vi "playback shoulder.vi"(4 "Home":bool, 5 "Rewind":bool, 7 "Playback":bool, 8 "Taper Limit":dbl=1.0, 9 "Playback allow":bool=TRUE, 10 "Encoder Recording Data":cluster{dbl, u32}[](array[cluster])=[{0.0, 20}, {0.0, 41}, {0.0, 60}, {0.0, 80}, {0.0, 100}, {0.0, 120}, {0.0, 141}, {0.0, 160}, {0.0, 180}, {0.0, 200}, {0.0, 220}, {0.0, 244}, {0.0, 263}, {0.0, 283}, {0.0, 303}, {0.0, 322}, {0.0, 343}, {0.0, 364}, {0.0, 385}, {0.0, 406}, {0.0, 421}, {0.0, 442}, {0.0, 465}, {0.0, 486}, {0.0, 510}, {0.0, 527}, {0.0, 547}, {0.0, 567}, {0.0, 586}, {0.0, 606}, {0.0, 626}, {0.0, 649}, {0.0, 669}, {0.0, 689}, {0.0, 709}, {0.0, 730}, {0.0, 750}, {0.0, 769}, {0.0, 789}, {0.0, 809}, {0.0, 830}, {0.0, 849}, {0.0, 870}, {0.0, 891}, {0.0, 911}, {0.0, 931}, {0.0, 953}, {0.0, 974}, {0.0, 993}, {0.0, 1013}, {0.0, 1032}, {0.0, 1052}, {0.0, 1073}, {0.0, 1093}, {0.0, 1114}, {0.0, 1134}, {0.0, 1155}, {0.0, 1174}, {0.0, 1194}, {0.0, 1214}, {0.0, 1235}, {0.0, 1255}, {0.0, 1275}, {0.0, 1297}, {0.0, 1317}, {0.0, 1337}, {0.0, 1357}, {0.0, 1379}, {0.0, 1399}, {0.0, 1417}, {0.0, 1438}, {0.0, 1458}, {0.0, 1479}, {0.0, 1499}, {0.0, 1519}, {0.0, 1540}, {0.0, 1560}, {0.0, 1579}, {0.0, 1600}, {0.0, 1619}, {0.0, 1639}, {0.0, 1660}, {0.0, 1679}, {0.0, 1699}, {0.0, 1720}, {0.0, 1741}, {0.0, 1760}, {0.0, 1787}, {0.0, 1801}, {0.0, 1823}, {0.0, 1841}, {0.0, 1864}, {0.0, 1884}, {0.0, 1904}, {0.0, 1925}, {0.0, 1945}, {0.0, 1966}, {0.0, 1986}, {0.0, 2006}, {0.0, 2028}, {0.0, 2047}, {0.0, 2068}, {0.0, 2087}, {0.0, 2107}, {0.0, 2128}, {0.0, 2147}, {0.0, 2167}, {0.0, 2189}, {0.0, 2208}, {0.0, 2227}, {0.0, 2248}, {0.0, 2268}, {0.0, 2288}, {0.0, 2308}, {0.0, 2329}, {0.0, 2348}, {0.0, 2369}, {0.0, 2389}, {0.0, 2408}, {0.0, 2429}, {0.0, 2448}, {-0.25, 2469}, {-1.0, 2488}, {-2.0, 2508}, {-2.75, 2529}, {-4.0, 2550}, {-4.5, 2570}, {-4.75, 2590}, {-5.0, 2610}, {-5.0, 2630}, {-5.25, 2651}, {-6.0, 2674}, {-7.0, 2693}, {-7.0, 2712}, {-7.25, 2734}, {-7.25, 2755}, {-7.25, 2775}, {-7.25, 2795}, {-7.5, 2815}, {-7.5, 2836}, {-8.0, 2855}, {-8.25, 2875}, {-8.75, 2896}, {-9.5, 2917}, {-9.75, 2937}, {-10.25, 2957}, {-10.75, 2977}, {-11.0, 2997}, {-11.5, 3016}, {-12.25, 3037}, {-13.25, 3058}, {-14.0, 3077}, {-15.0, 3097}, {-16.25, 3117}, {-17.5, 3137}, {-18.75, 3157}, {-20.0, 3178}, {-21.5, 3198}, {-23.0, 3218}, {-24.5, 3238}, {-26.0, 3258}, {-27.5, 3278}, {-28.75, 3298}, {-30.25, 3318}, {-31.25, 3339}, {-32.0, 3359}, {-32.25, 3380}, {-32.75, 3400}, {-33.25, 3419}, {-34.5, 3444}, {-35.0, 3461}, {-35.5, 3481}, {-36.0, 3501}, {-36.25, 3521}, {-36.75, 3541}, {-37.25, 3560}, {-38.0, 3581}, {-39.0, 3600}, {-40.25, 3620}, {-41.75, 3641}, {-43.25, 3661}, {-45.25, 3680}, {-48.0, 3704}, {-49.75, 3720}, {-52.0, 3741}, {-54.75, 3762}, {-57.5, 3782}, {-61.0, 3806}, {-63.5, 3822}, {-67.0, 3844}, {-70.25, 3865}, {-73.0, 3886}, {-75.75, 3904}, {-78.5, 3926}, {-81.0, 3945}, {-83.5, 3965}, {-86.25, 3986}, {-89.0, 4006}, {-91.75, 4026}, {-94.75, 4046}, {-97.75, 4066}, {-101.25, 4087}, {-105.5, 4108}, {-109.5, 4128}, {-113.75, 4149}, {-118.5, 4169}, {-123.5, 4190}, {-127.75, 4209}, {-132.75, 4229}, {-137.75, 4249}, {-142.5, 4269}, {-147.25, 4289}, {-151.75, 4309}, {-156.25, 4329}, {-160.75, 4349}, {-165.25, 4369}, {-169.5, 4389}, {-173.75, 4409}, {-178.0, 4429}, {-182.25, 4449}, {-186.5, 4469}, {-191.25, 4490}, {-195.75, 4510}, {-200.25, 4529}, {-205.0, 4549}, {-210.25, 4570}, {-215.25, 4590}, {-220.25, 4609}, {-225.75, 4629}, {-230.75, 4650}, {-235.75, 4669}, {-241.25, 4690}, {-246.5, 4710}, {-251.75, 4731}, {-257.0, 4751}, {-261.75, 4770}, {-266.75, 4791}, {-271.75, 4811}, {-276.5, 4830}, {-282.0, 4854}, {-286.5, 4873}, {-292.0, 4894}, {-296.25, 4910}, {-301.25, 4931}, {-306.25, 4950}, {-311.25, 4970}, {-317.0, 4993}, {-322.25, 5013}, {-327.25, 5033}, {-332.25, 5053}, {-337.25, 5073}, {-342.25, 5093}, {-346.5, 5112}, {-351.5, 5133}, {-356.0, 5153}, {-360.5, 5173}, {-365.0, 5193}, {-369.5, 5213}, {-373.75, 5233}, {-378.75, 5256}, {-383.25, 5277}, {-387.5, 5295}, {-391.5, 5314}, {-396.0, 5334}, {-400.5, 5354}, {-405.25, 5376}, {-410.0, 5396}, {-414.25, 5415}, {-419.0, 5435}, {-423.5, 5454}, {-428.0, 5474}, {-432.5, 5495}, {-437.0, 5516}, {-441.25, 5534}, {-445.75, 5555}, {-450.25, 5576}, {-454.5, 5594}, {-458.5, 5615}, {-462.5, 5634}, {-466.5, 5654}, {-471.25, 5677}, {-475.75, 5698}, {-479.5, 5717}, {-484.0, 5738}, {-488.25, 5758}, {-492.25, 5779}, {-496.75, 5799}, {-500.75, 5820}, {-504.75, 5839}, {-509.0, 5859}, {-513.0, 5878}, {-517.25, 5899}, {-521.25, 5918}, {-525.5, 5938}, {-529.5, 5958}, {-533.75, 5979}, {-537.75, 5999}, {-541.5, 6019}, {-545.5, 6039}, {-549.25, 6059}, {-553.25, 6079}, {-556.75, 6098}, {-560.75, 6120}, {-564.25, 6138}, {-568.0, 6159}, {-571.75, 6179}, {-575.5, 6200}, {-579.0, 6219}, {-582.75, 6240}, {-586.5, 6261}, {-590.0, 6280}, {-593.75, 6300}, {-597.5, 6321}, {-600.75, 6339}, {-604.5, 6360}, {-608.25, 6381}, {-611.75, 6399}, {-615.25, 6419}, {-619.0, 6439}, {-623.25, 6462}, {-626.75, 6480}, {-630.5, 6500}, {-634.25, 6519}, {-638.25, 6540}, {-642.0, 6559}, {-646.5, 6581}, {-650.5, 6600}, {-654.75, 6620}, {-658.75, 6639}, {-663.0, 6660}, {-667.25, 6679}, {-671.75, 6699}, {-676.25, 6720}, {-680.75, 6740}, {-685.25, 6761}, {-690.0, 6782}, {-694.25, 6802}, {-699.0, 6822}, {-704.25, 6847}, {-709.0, 6867}, {-713.25, 6887}, {-717.75, 6907}, {-722.25, 6927}, {-727.0, 6949}, {-731.75, 6970}, {-736.5, 6991}, {-741.0, 7011}, {-745.75, 7031}, {-750.75, 7051}, {-756.25, 7074}, {-760.5, 7092}, {-765.0, 7111}, {-770.75, 7133}, {-774.75, 7150}, {-780.25, 7173}, {-785.25, 7194}, {-790.25, 7214}, {-795.0, 7235}, {-799.75, 7255}, {-804.75, 7276}, {-809.0, 7295}, {-814.0, 7316}, {-819.0, 7338}, {-823.5, 7357}, {-828.0, 7377}, {-832.5, 7398}, {-837.0, 7419}, {-841.25, 7438}, {-845.75, 7459}, {-850.25, 7480}, {-854.5, 7500}, {-858.75, 7521}, {-863.0, 7541}, {-867.5, 7563}, {-871.5, 7582}, {-875.75, 7603}, {-880.0, 7624}, {-884.0, 7644}, {-888.25, 7666}, {-892.5, 7687}, {-896.0, 7704}, {-900.0, 7725}, {-903.5, 7744}, {-907.75, 7765}, {-911.5, 7786}, {-915.5, 7806}, {-918.75, 7825}, {-923.0, 7845}, {-926.75, 7865}, {-930.25, 7886}, {-933.75, 7907}, {-937.5, 7928}, {-940.75, 7947}, {-944.0, 7968}, {-947.25, 7990}, {-949.75, 8006}, {-953.0, 8027}, {-956.0, 8048}, {-958.75, 8068}, {-961.25, 8087}, {-964.0, 8108}, {-966.5, 8128}, {-969.0, 8148}, {-971.0, 8167}, {-973.75, 8190}, {-975.75, 8208}, {-978.0, 8230}, {-980.0, 8250}, {-981.75, 8269}, {-984.0, 8291}, {-986.0, 8312}, {-988.0, 8332}, {-989.5, 8349}, {-991.5, 8373}, {-992.75, 8391}, {-994.0, 8410}, {-995.5, 8431}, {-996.75, 8451}, {-998.0, 8474}, {-999.25, 8494}, {-1000.25, 8514}, {-1001.5, 8535}, {-1002.5, 8557}, {-1003.5, 8577}, {-1004.75, 8595}, {-1006.0, 8615}, {-1007.25, 8634}, {-1008.75, 8657}, {-1010.0, 8676}, {-1011.5, 8697}, {-1013.0, 8717}, {-1014.25, 8736}, {-1015.5, 8756}, {-1016.75, 8777}, {-1017.25, 8798}, {-1017.25, 8817}, {-1017.5, 8837}, {-1017.5, 8857}, {-1017.75, 8880}, {-1018.0, 8895}, {-1018.5, 8918}, {-1019.25, 8937}, {-1020.25, 8957}, {-1021.25, 8979}, {-1021.5, 9006}, {-1021.5, 9018}, {-1021.75, 9042}, {-1022.0, 9057}, {-1022.5, 9078}, {-1023.75, 9106}, {-1024.5, 9120}, {-1026.0, 9139}, {-1027.75, 9159}, {-1029.75, 9179}, {-1031.75, 9199}, {-1034.5, 9220}, {-1036.75, 9239}, {-1039.75, 9259}, {-1042.75, 9278}, {-1045.75, 9299}, {-1049.5, 9319}, {-1052.75, 9338}, {-1055.75, 9358}, {-1058.5, 9378}, {-1061.25, 9399}, {-1063.5, 9418}, {-1066.25, 9438}, {-1068.75, 9458}, {-1071.0, 9479}, {-1073.25, 9498}, {-1075.5, 9519}, {-1077.5, 9538}, {-1079.75, 9559}, {-1082.25, 9582}, {-1084.75, 9603}, {-1087.25, 9621}, {-1090.25, 9644}, {-1093.0, 9662}, {-1096.5, 9685}, {-1099.5, 9705}, {-1102.25, 9723}, {-1105.5, 9745}, {-1108.5, 9764}, {-1112.75, 9790}, {-1115.75, 9809}, {-1118.75, 9830}, {-1121.75, 9851}, {-1124.5, 9870}, {-1127.25, 9890}, {-1130.0, 9909}, {-1132.75, 9931}, {-1135.25, 9949}, {-1138.0, 9970}, {-1140.75, 9991}, {-1143.0, 10009}, {-1145.5, 10029}, {-1148.25, 10050}, {-1151.5, 10073}, {-1154.0, 10090}, {-1157.0, 10110}, {-1159.75, 10130}, {-1163.0, 10150}, {-1166.25, 10172}, {-1170.0, 10194}, {-1173.25, 10215}, {-1176.25, 10235}, {-1179.25, 10254}, {-1182.25, 10275}, {-1185.5, 10297}, {-1188.0, 10315}, {-1190.75, 10336}, {-1193.5, 10356}, {-1196.0, 10376}, {-1198.25, 10395}, {-1200.75, 10416}, {-1202.75, 10437}, {-1205.0, 10456}, {-1207.0, 10476}, {-1209.0, 10497}, {-1211.0, 10517}, {-1213.0, 10536}, {-1215.0, 10556}, {-1216.75, 10577}, {-1218.75, 10597}, {-1220.5, 10617}, {-1222.5, 10638}, {-1224.0, 10658}, {-1225.75, 10678}, {-1227.25, 10699}, {-1229.0, 10720}, {-1230.25, 10738}, {-1232.0, 10759}, {-1233.5, 10780}, {-1235.0, 10799}, {-1236.5, 10819}, {-1238.0, 10839}, {-1239.25, 10858}, {-1240.75, 10879}, {-1242.5, 10901}, {-1243.75, 10919}, {-1245.5, 10940}, {-1247.0, 10960}, {-1248.5, 10979}, {-1250.25, 11000}, {-1251.75, 11020}, {-1253.25, 11041}, {-1254.75, 11060}, {-1256.5, 11081}, {-1257.75, 11099}, {-1259.75, 11123}, {-1261.0, 11140}, {-1262.25, 11159}, {-1263.75, 11180}, {-1265.0, 11200}, {-1266.75, 11220}, {-1268.0, 11239}, {-1269.75, 11259}, {-1271.25, 11280}, {-1272.75, 11299}, {-1274.5, 11320}, {-1276.25, 11340}, {-1278.0, 11364}, {-1279.5, 11381}, {-1281.25, 11401}, {-1283.25, 11424}, {-1284.5, 11441}, {-1286.0, 11462}, {-1287.5, 11485}, {-1288.25, 11500}, {-1289.75, 11521}, {-1290.75, 11540}, {-1291.75, 11563}, {-1292.75, 11581}, {-1293.75, 11601}, {-1294.5, 11621}, {-1295.5, 11643}, {-1296.25, 11661}, {-1297.25, 11682}, {-1298.25, 11704}, {-1299.0, 11724}, {-1300.25, 11744}, {-1301.25, 11764}, {-1302.75, 11783}, {-1304.0, 11802}], 11 "Hardware In":T5={"Motor Selection"="Shoulder", "EncoderDevRef"={"DevStatus"={"status"=FALSE, "code"=0, "source"=""}, "EncoderIndex"=enum."Enc 1", "CounterIndex"=enum."Invalid", "DistancePerCount"=1.0, "Decoding Type"=enum."4x"}}) -> (0 "Encoder Distance PB":dbl)   [LabVIEW 2017]
uses:
  <vilib>/Rock Robotics/WPI/Encoder/WPI_EncoderDevRef.ctl
  <vilib>/Rock Robotics/SystemInterfaces/Encoder/FPGA_EncoderIdx.ctl
  <vilib>/Rock Robotics/SystemInterfaces/Counter/FPGA_CounterCtrSystemIndex.ctl
  <vilib>/Rock Robotics/WPI/Encoder/WPI_EncoderType.ctl
  <vilib>/Rock Robotics/WPI/Utilities/WPI_GetSetVariantRefNum.vi
  <vilib>/addons/control/pid/pid.llb/PID (DBL).vi
  <vilib>/Rock Robotics/WPI/RobotDrive/WPI_RobotDriveArcadeDrive_Standard(NoSaturation).vi
  <vilib>/addons/control/pid/NI_PID_pid.lvlib
panel:
  out "Initial Encoder Position":dbl=-58.0
  out "Waveform Chart":cluster{dbl, dbl}(graph)={0.0, -2.0}
  in  "Playback PID gains":T6={"proportional gain (Kc)"=-0.015, "integral time (Ti, min)"=0.014, "derivative time (Td, min)"=0.0} {"derivative time (Td, min)" format="%.8f"; "integral time (Ti, min)" format="%.8f"; "proportional gain (Kc)" format="%.8f"}
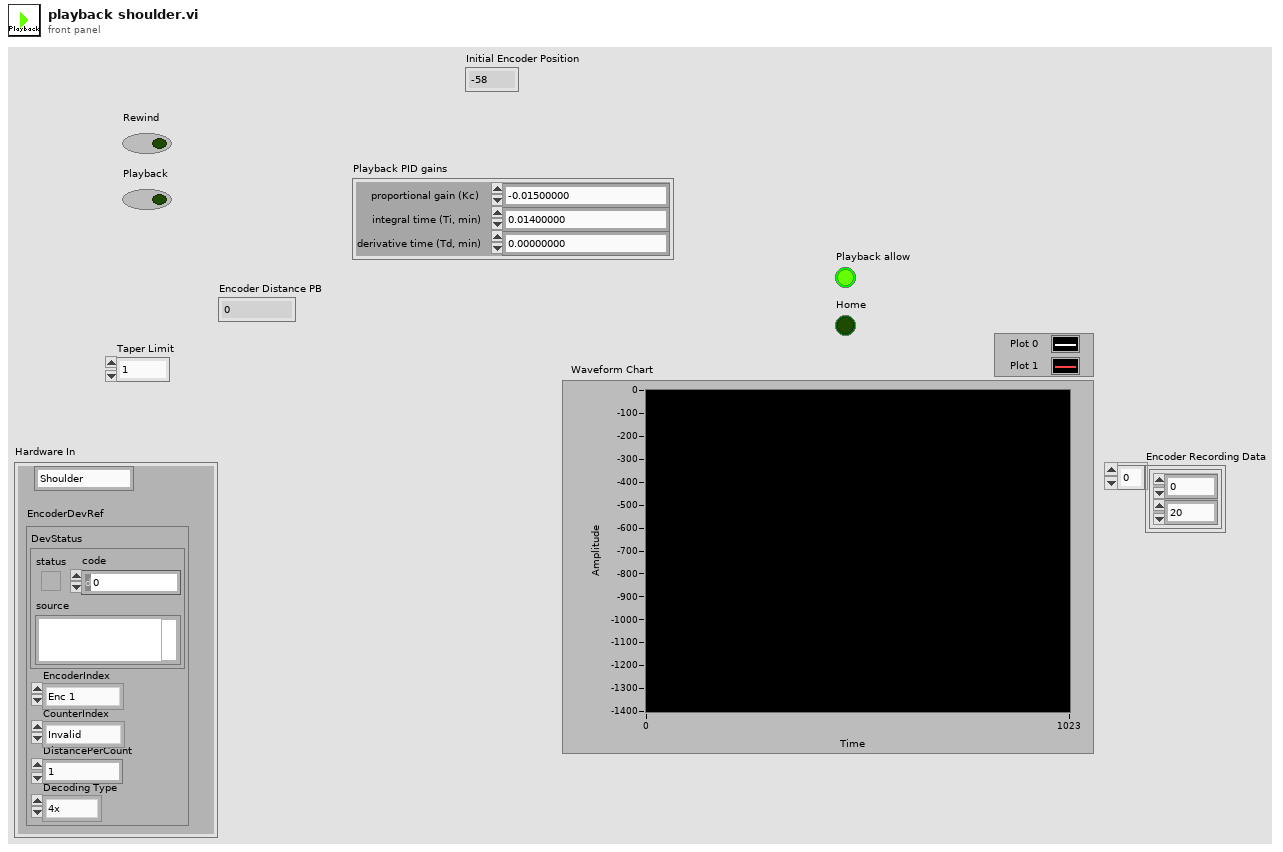
[diagram p1: front panel]
types:
  T1 = typedef "WPI_EncoderDevRef.ctl" = cluster{"DevStatus":errorcluster, "EncoderIndex":T2, "CounterIndex":T3, "DistancePerCount":dbl, "Decoding Type":T4}
  T2 = typedef "FPGA_EncoderIdx.ctl" = enum8{"Enc 0", "Enc 1", "Enc 2", "Enc 3", "Enc 4", "Enc 5", "Enc 6", "Enc 7", "Invalid"}
  T3 = typedef "FPGA_CounterCtrSystemIndex.ctl" = enum8{"Ctr 0", "Ctr 1", "Ctr 2", "Ctr 3", "Ctr 4", "Ctr 5", "Ctr 6", "Ctr 7", "Invalid"}
  T4 = typedef "WPI_EncoderType.ctl" = enum16{"1x", "2x", "4x"}
  T5 = cluster{"Motor Selection":string, "EncoderDevRef":T1}
  T6 = cluster{"proportional gain (Kc)":dbl, "integral time (Ti, min)":dbl, "derivative time (Td, min)":dbl}
  T7 = typedef "WPI_RobotDriveDevRef.ctl" = cluster{"DevStatus":errorcluster, "Motors[]":T8[], "Square Inputs":bool, "Max Output":dbl}
  T8 = typedef "WPI_MotorControlDeviceRef.ctl" = cluster{"DeviceStatus":errorcluster, "Type":T9, "PWM":cluster{"PWM Channel":T10, "DeadBand":T11}, "CAN":cluster{"Device Number":u8, "SetOutput VI Ref":variant, "GetOutput VI Ref":variant, "Enable VI Ref":variant, "Disable VI Ref":variant, "Data":variant}, "Invert":bool, "DIO PWM":cluster{"PWM \"Enable\" Channel":T10, "DIOChannel":T12, "PWM Rate":dbl}}
  T9 = typedef "WPI_MotorControlType.ctl" = enum16{"PWM", "CAN", "DIO PWM"}
  T10 = typedef "FPGA_DIOPWMChannel.ctl" = enum8{"PWM 0", "PWM 1", "PWM 2", "PWM 3", "PWM 4", "PWM 5", "PWM 6", "PWM 7", "PWM 8", "PWM 9", "PWM MXP 0", "PWM MXP 1", "PWM MXP 2", "PWM MXP 3", "PWM MXP 4", "PWM MXP 5", "PWM MXP 6", "PWM MXP 7", "PWM MXP 8", "PWM MXP 9", "Invalid"}
  T11 = typedef "WPI_PWMDeadband.ctl" = cluster{"Name":string, "maxPositivePwm":i32, "minPositivePwm":i32, "centerPwm":i32, "maxNegativePwm":i32, "minNegativePwm":i32, "angularRange":u16}
  T12 = typedef "FPGA_DIOChannel.ctl" = enum8{"DIO 0", "DIO 1", "DIO 2", "DIO 3", "DIO 4", "DIO 5", "DIO 6", "DIO 7", "DIO 8", "DIO 9", "DIO MXP 0", "DIO MXP 1", "DIO MXP 2", "DIO MXP 3", "DIO MXP 4", "DIO MXP 5", "DIO MXP 6", "DIO MXP 7", "DIO MXP 8", "DIO MXP 9", "DIO MXP 10", "DIO MXP 11", "DIO MXP 12", "DIO MXP 13", "DIO MXP 14", "DIO MXP 15", "SPI Port CS1", "SPI Port CS2", "SPI Port CS3", "SPI Port MISO", "SPI Port MOSI", "Invalid"}
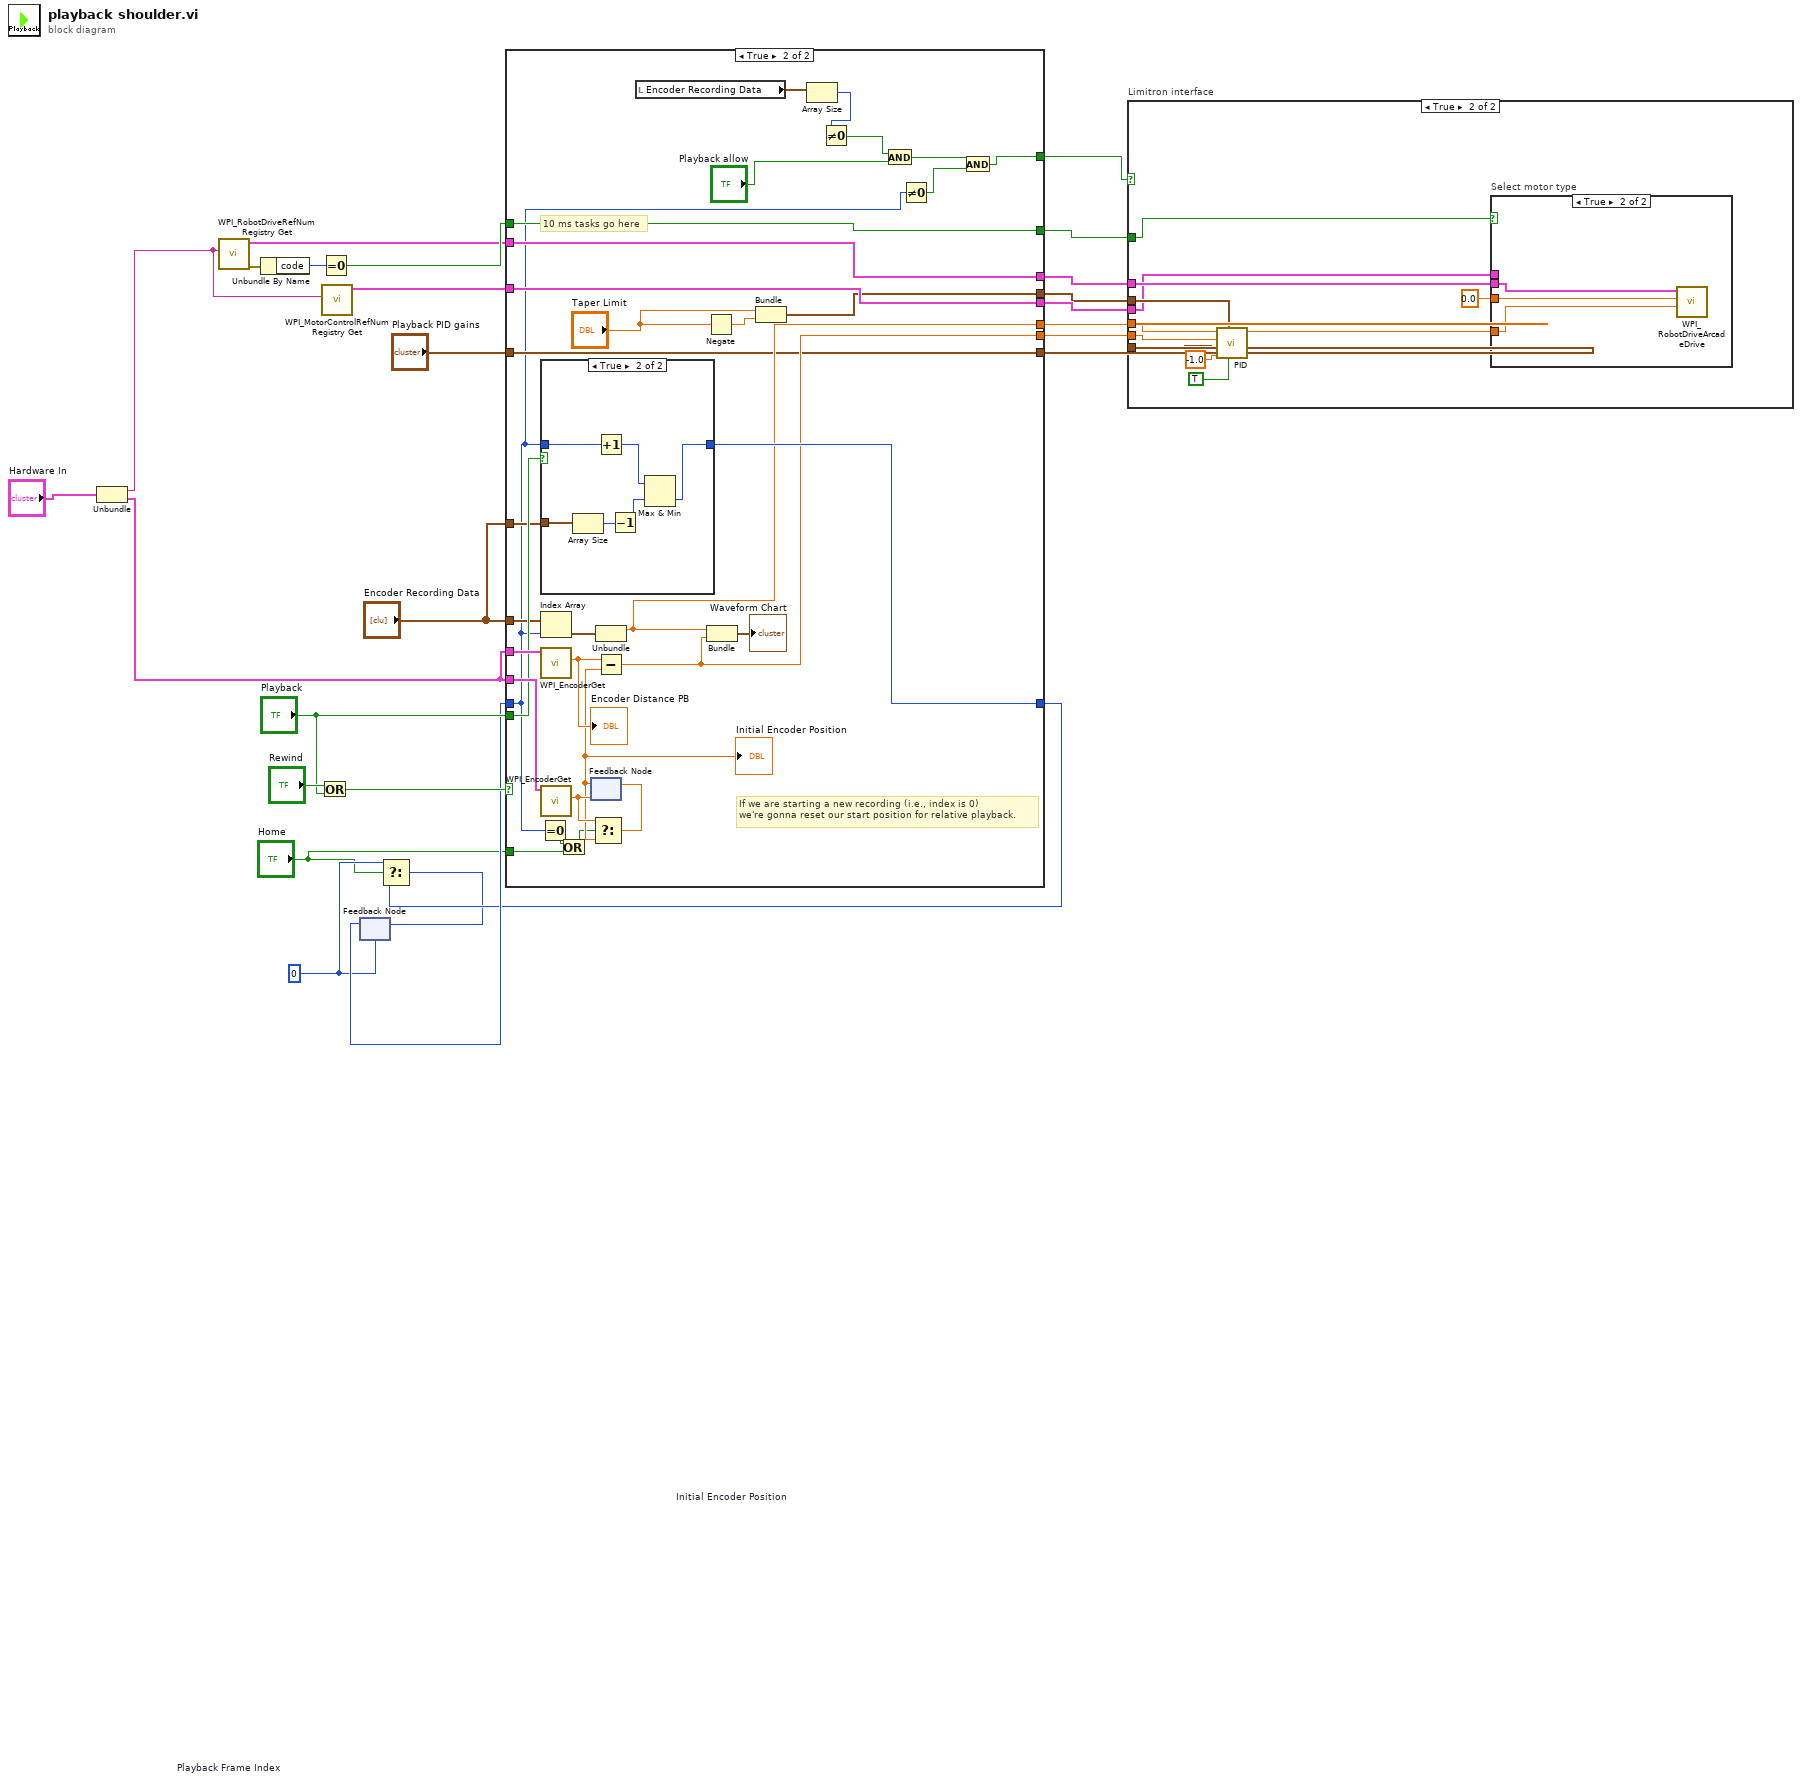
[diagram p0: block diagram]
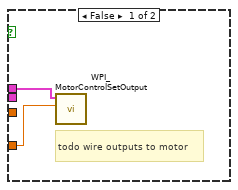
[diagram p3: hidden frame]
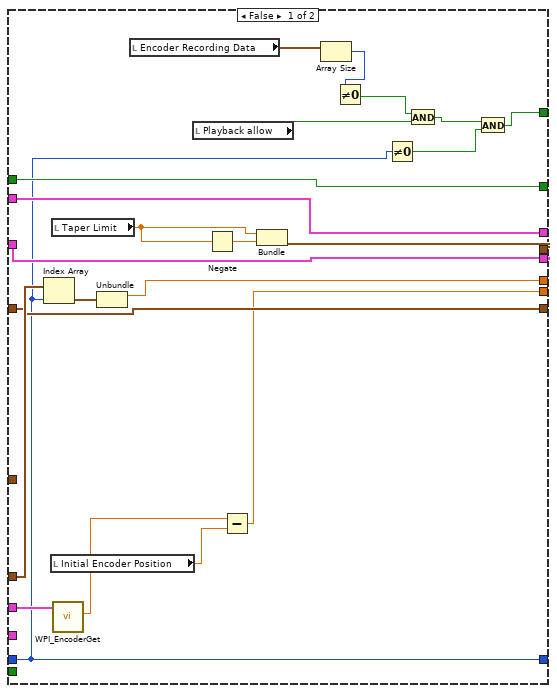
[diagram p4: hidden frame]
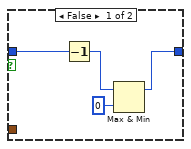
[diagram p5: hidden frame]
diagram:
  w15 = 0 ("index")
  n1 = Unbundle("Hardware In") -> ("Motor Selection"=w11:string, "EncoderDevRef"=w10:T1)
  n2 = call <vilib>:"WPI_RobotDriveRefNum Registry Get.vi"("refnum name"=w11) -> ("error out"=w25:errorcluster, "RobotDriveDevRef"=w23:T7)  [unwired: 1 in, 8 out]
  n3 = Unbundle By Name(w25) -> ("code"=w26:i32)
  n4 = Or(x="Rewind", y="Playback") -> (x .or. y?=w21:bool)
  n5 = Equal To 0?(x=w26) -> (x = 0?=w24:bool)
  n6 = call <vilib>:"WPI_MotorControlRefNum Registry Get.vi"("refnum name"=w11) -> ("MotorControlDevRef"=w19:T8)  [unwired: 9 in, 1 out]
  n7 = feedback #1 "Playback Frame Index"(w15) -> (w18:i32)
  n8 = case shown="True" w21 {
    tunnel: w10 -> [_ w80]
    tunnel: w10 -> [w34 w79]
    tunnel: w24 -> [w44 w67]
    tunnel: w23 -> [w43 w66]
    tunnel: "Playback" -> [_ w78]
    tunnel: w19 -> [w42 w65]
    tunnel: "Encoder Recording Data" -> [w48 w72]
    tunnel: w18 -> [w27 w52]
    tunnel: [w27 w71] -> w16
    tunnel: "Playback PID gains" -> [w40 w61]
    tunnel: "Encoder Recording Data" -> [_ w68]
    tunnel: [w44 w67] -> w9
    tunnel: [w43 w66] -> w8
    tunnel: [w42 w65] -> w7
    tunnel: [w41 w64] -> w6
    tunnel: [w31 w63] -> w5
    tunnel: [w39 w62] -> w4
    tunnel: [w40 w61] -> w3
    tunnel: [w28 w54] -> w2
    tunnel: "Home" -> [_ w49]
    frame False {
      n9 = Index Array(array=w48, index=w27) -> (element=w47:cluster{dbl, u32})
      n10 = local read "Initial Encoder Position"() -> (w32:dbl)
      n11 = local read "Taper Limit"() -> (w45:dbl)
      n12 = call <vilib>:"WPI_EncoderGet.vi"("EncoderDevRef"=w34) -> ("Distance"=w33:dbl)  [unwired: 5 in, 5 out]
      n13 = Unbundle(w47) -> (w41:dbl)  [unwired: 1 out]
      n14 = local read "Encoder Recording Data"() -> (w35:cluster{dbl, u32}[])
      n15 = local read "Playback allow"() -> (w36:bool)
      n16 = Negate(x=w45) -> (-x=w46:dbl)
      n17 = Subtract(x=w33, y=w32) -> (x-y=w31:dbl)
      n18 = Bundle("Taper Limit"=w45, w46) -> (w39:cluster{"Taper Limit":dbl, dbl})  [unwired: 1 in]
      n19 = Array Size(array=w35) -> (size(s)=w38:i32)
      n20 = Not Equal To 0?(x=w38) -> (x != 0?=w37:bool)
      n21 = Not Equal To 0?(x=w27) -> (x != 0?=w29:bool)
      n22 = And(x=w37, y=w36) -> (x .and. y?=w30:bool)
      n23 = And(x=w30, y=w29) -> (x .and. y?=w28:bool)
    }
    frame True {
      # "If we are starting a new recording (i.e., index is 0)\nwe're gonna reset our start position for relative playback."
      # "10 ms tasks go here"
      n24 = Equal To 0?(x=w52) -> (x = 0?=w50:bool)
      n25 = case shown="True" w78 {
        tunnel: [w81 w88] -> w71
        tunnel: w52 -> [w84 w90]
        tunnel: w68 -> [_ w87]
        frame False {
          n26 = Decrement(x=w84) -> (x-1=w82:i32)
          n27 = Max & Min(x=w82, y=0) -> (max(x,y)=w81:i32)  [unwired: 1 out]
        }
        frame True {
          n28 = Array Size(array=w87) -> (size(s)=w86:i32)
          n29 = Increment(x=w90) -> (x+1=w89:i32)
          n30 = Decrement(x=w86) -> (x-1=w85:i32)
          n31 = Max & Min(x=w89, y=w85) -> (min(x,y)=w88:i32)  [unwired: 1 out]
        }
      }
      n32 = Index Array(array=w72, index=w52) -> (element=w73:cluster{dbl, u32})
      n33 = call <vilib>:"WPI_EncoderGet.vi"("EncoderDevRef"=w79) -> ("Distance"=w77:dbl)  [unwired: 5 in, 5 out]
      "Encoder Distance PB" <- w77
      n34 = call <vilib>:"WPI_EncoderGet.vi"("EncoderDevRef"=w80) -> ("Distance"=w70:dbl)  [unwired: 5 in, 5 out]
      n35 = Or(x=w50, y=w49) -> (x .or. y?=w51:bool)
      n36 = feedback #2 "Initial Encoder Position"(w70) -> (w69:dbl)
      "Initial Encoder Position" <- w69
      n37 = Select(t=w70, s=w51, f=w69) -> (s? t:f=w56:dbl)
      n38 = feedback-in #2(w56) -> ()
      n39 = Unbundle(w73) -> (w64:dbl)  [unwired: 1 out]
      n40 = Subtract(x=w77, y=w69) -> (x-y=w63:dbl)
      n41 = local read "Encoder Recording Data"() -> (w59:cluster{dbl, u32}[])
      n42 = Negate(x="Taper Limit") -> (-x=w75:dbl)
      n43 = Bundle(w64, w63) -> (→"Waveform Chart":cluster{dbl, dbl})  [unwired: 1 in]
      n44 = Bundle("Taper Limit"="Taper Limit", w75) -> (w62:cluster{"Taper Limit":dbl, dbl})  [unwired: 1 in]
      n45 = Array Size(array=w59) -> (size(s)=w60:i32)
      n46 = Not Equal To 0?(x=w60) -> (x != 0?=w57:bool)
      n47 = And(x=w57, y="Playback allow") -> (x .and. y?=w55:bool)
      n48 = Not Equal To 0?(x=w52) -> (x != 0?=w53:bool)
      n49 = And(x=w55, y=w53) -> (x .and. y?=w54:bool)
    }
  }
  n50 = Select(t=w15, s="Home", f=w16) -> (s? t:f=w14:i32)
  n51 = feedback-in #1(w14) -> ()
  n52 = case "Limitron interface" shown="True" w2 {
    tunnel: w3 -> [_ w101]
    tunnel: w5 -> [_ w98]
    tunnel: w6 -> [_ w97]
    tunnel: w7 -> [_ w92]
    tunnel: w9 -> [_ w93]
    tunnel: w8 -> [_ w95]
    tunnel: w4 -> [_ w94]
    frame False {
    }
    frame True {
      n53 = call-poly <vilib>:"PID.vi"("reinitialize? (F)"=TRUE, "output range"=w94, "dt (s)"=-1.0, "PID gains"=w101, "process variable"=w98, "setpoint"=w97) -> ("output"=w96:dbl)  [unwired: 4 in, 1 out]
      n54 = case "Select motor type" shown="True" w93 {
        tunnel: 0.0 ("output") -> [_ w106]
        tunnel: w96 -> [w103 w105]
        tunnel: w95 -> [_ w104]
        tunnel: w92 -> [w102 _]
        frame False {
          # "todo wire outputs to motor"
          n55 = call <vilib>:"WPI_MotorControlSetOutput.vi"("Output"=w103, "MotorControlDevRef"=w102) -> ()  [unwired: 7 in, 3 out]
        }
        frame True {
          n56 = call-poly <vilib>:"WPI_RobotDriveArcadeDrive.vi"("Y axis value"=w105, "X axis value"=w106, "RobotDriveDevRef"=w104) -> ()  [unwired: 6 in, 3 out]
        }
      }
    }
  }
